vi "Connect.vi"(8 "Error In":errorcluster, 10 "Resource Name":refnum<k15>, 11 "object in":refnum<class "Error.lvclass">) -> (0 "Error Out":errorcluster, 2 "Resource Name out":refnum<k15>, 3 "object out":refnum<class "IStates.lvclass">)   [LabVIEW 2023, in "PXI-5441.lvlib" / "Error.lvclass"]
uses:
  Error.lvclass
  IScope_interface/IStates_interface/IStates.lvclass
  Error.lvclass/Error.ctl
  D:/git/HAL/PXI-5441_class/states/Error_class/Error.lvclass
  D:/git/HAL/IScope_interface/IStates_interface/IStates.lvclass
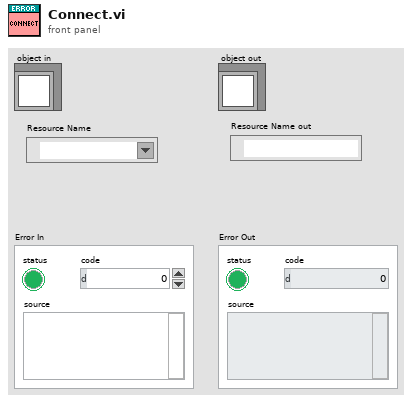
[diagram p1: front panel]
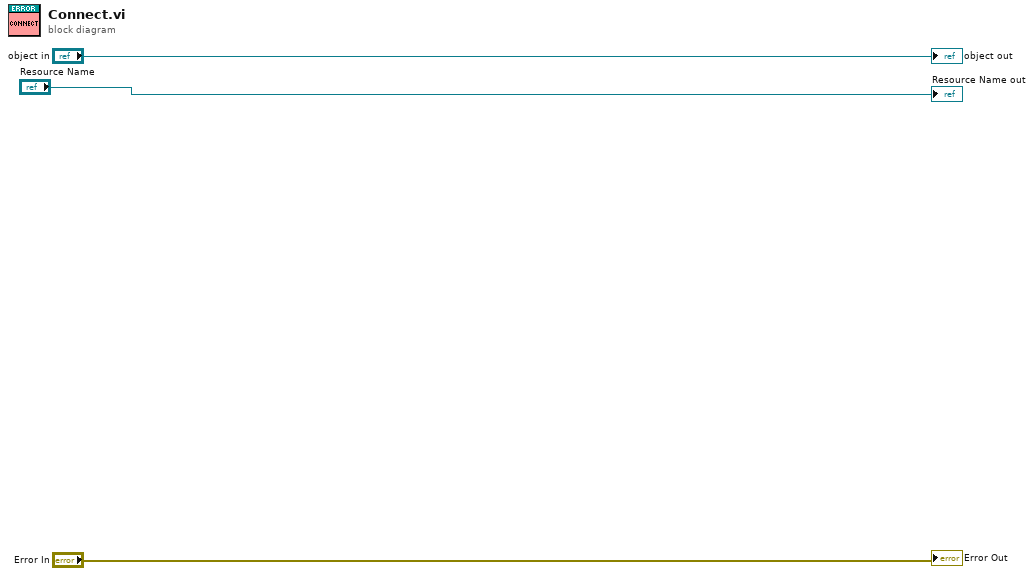
[diagram p0: block diagram]
diagram:
  "Error Out" <- "Error In"
  "object out" <- "object in"
  "Resource Name out" <- "Resource Name"
